vi "836_Drive_Train.vi"   [LabVIEW 2015]
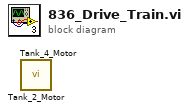
[diagram p0: block diagram]
diagram:
  n1 = call <userlib>:"Tank_2_Motor.vi"() -> ()  [unwired: 11 in, 1 out]
  n2 = call <userlib>:"Tank_4_Motor.vi"() -> ()  [unwired: 11 in, 1 out]
